vi "Display Tree on GUI.vi"(8 "error in (no error)":errorcluster, 10 "Tree on GUI":refnum<vi>, 11 "Data":refnum<vi>) -> (0 "error out":errorcluster)   [LabVIEW 2021, in "CANOpen Addon System Explorer.lvlib"]
uses:
  CANOpen Addon System Explorer.lvlib
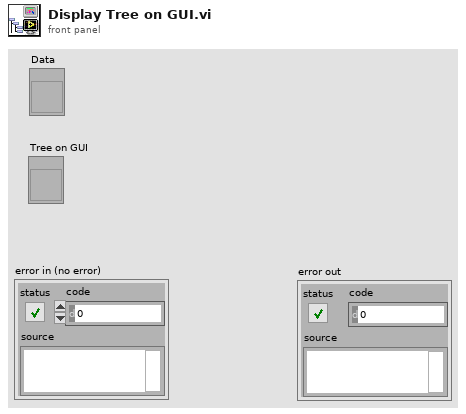
[diagram p1: front panel]
types:
  T1 = typedef "CANOpen Addon System Explorer.lvlib/OD Entry.ctl" = cluster{"index":u16, "sub-index":u8, "Level":u8, "ObjectType":T2, "DataType":T3, "ParameterName":string, "LowLimit":string, "HighLimit":string, "AccessType":T4, "DefaultValue":string, "PDOMapping":bool, "SubNumber":u8, "ObjFlags":u32, "Category":T5}
  T2 = typedef "CANOpen Addon System Explorer.lvlib/Object Type.ctl" = u16
  T3 = typedef "CANOpen Addon System Explorer.lvlib/Data Type.ctl" = u16
  T4 = typedef "CANOpen Addon System Explorer.lvlib/Access Type.ctl" = u16
  T5 = typedef "CANOpen Addon System Explorer.lvlib/OD Cateory.ctl" = enum16{"Mandatory", "Optional", "Manufacturer", ""}
  T6 = cluster{"Left Cell String":string, "Child Text":string[], "Child Tag":string, "Item Indent":i32, "Child Only?":bool, "Glyph Index":i32}
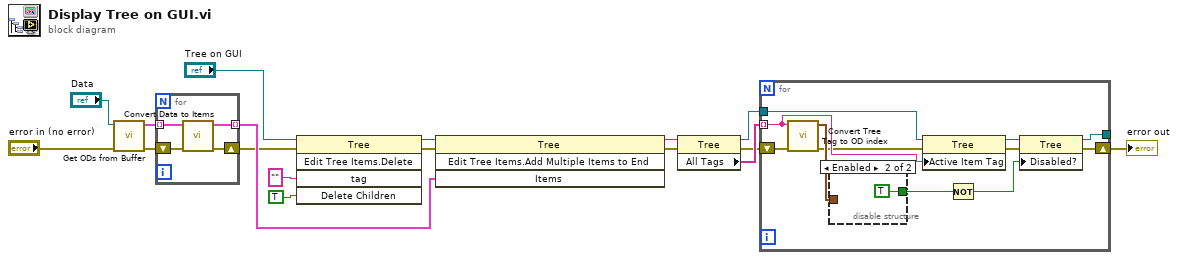
[diagram p0: block diagram]
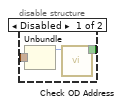
[diagram p2: hidden frame]
diagram:
  n1 = call "Get ODs from Buffer.vi"("error in (no error)"="error in (no error)", "Data"="Data") -> ("error out"=w10:errorcluster, "data"=w9:T1[])  [unwired: 8 in]
  n2 = for {
    shift-right: [w18] -> w3
    shift-left: w10 -> [w19]
    tunnel: w9 -> [w21] mode=indexing
    tunnel: [w20] -> w17 mode=indexing
    n3 = call "Convert Data to Items.vi"("error in"=w19, "OD Entry"=w21) -> ("error out"=w18:errorcluster, "Item"=w20:T6)  [unwired: 8 in]
  }
  n4 = invoke class="Tree" method="Edit Tree Items.Delete"(reference="Tree on GUI", error in=w3, "tag"="" ("Tag"), "Delete Children"=TRUE ("Delete Children?")) -> (reference out=w16:refnum<vi>, error out=w15:errorcluster)  [unwired: 1 in, 3 out]
  n5 = invoke class="Tree" method="Edit Tree Items.Add Multiple Items to End"(reference=w16, error in=w15, "Items"=w17) -> (reference out=w8:refnum<vi>, error out=w7:errorcluster)  [unwired: 1 in, 2 out]
  n6 = property class="Tree"(reference=w8, error in=w7) -> (reference out=w4:refnum<vi>, error out=w5:errorcluster, "All Tags"=w6:string[])
  n7 = for {
    tunnel: w6 -> [w31] mode=indexing
    tunnel: w4 -> [w32]
    shift-right: [w27] -> w1
    shift-left: w5 -> [w23]
    tunnel: [w24] -> _
    n8 = call "Convert Tree Tag to OD index.vi"("error in"=w23, "Tag"=w31) -> ("error out"=w22:errorcluster, "index"=w30:cluster{u16, u8, u8})  [unwired: 8 in]
    n9 = disable-structure shown="Enabled" {
      disable-tunnel: w30 -> [w35 _]
      disable-tunnel: [w33 TRUE ("Support?")] -> w26
      frame Disabled {
        n10 = Unbundle(w35) -> (w34:u16)  [unwired: 2 out]
        n11 = call "Check OD Address.vi"("Address"=w34) -> ("Support?"=w33:bool)  [unwired: 10 in]
      }
      frame Enabled {
      }
    }
    n12 = property class="Tree"(reference=w32, error in=w22, "Active Item Tag"=w31) -> (reference out=w28:refnum<vi>, error out=w29:errorcluster)
    n13 = Not(x=w26) -> (.not. x?=w25:bool)
    n14 = property class="Tree"(reference=w28, error in=w29, "Disabled?"=w25) -> (reference out=w24:refnum<vi>, error out=w27:errorcluster)
  }
  "error out" <- w1
